vi "Acquire.vi"(8 "error in (no error)":errorcluster, 9 "Data Queue":refnum<queue>, 10 "Data Notifier":refnum<notifier>, 11 "Hardware Resources in":T1={"VISA resource name"="", "DAQ Type"=0, "Channel 1"={"Acquiring"=FALSE, "Enabled"=FALSE, "Terminal configuration"=32767, "Range"=0, "Coupling"=0}, "Channel 2"={"Acquiring"=FALSE, "Enabled"=FALSE, "Terminal configuration"=0, "Range"=0, "Coupling"=0}, "Timing"={"Sample Time [Time Units]"=0, "Actual Sample Time [s]"=0.0, "Samples per Iteration"=0, "Sample Clock Source"=0, "Time Units"=0, "t0"=timestamp(0 s since 1904-01-01)}, "PS Parameters"={"PS handle"=0, "PS Max_adc"=32767, "PS Enabled Array"=[], "PS Device Info"={"Driver Version"="", "USB Version"="", "Hardware"="", "Variant"="", "Batch and Serial"="", "Cal Date"="", "Kernel Version"="", "Digital HW Version"="", "Analogue HW Version"="", "Firmware 1"="", "Firmware 2"="", "MSO"=FALSE, "Number of Channels"=0}, "Channel 1 Buffer"=refnum, "Channel 2 Buffer"=refnum, "Resolution"=0, "USB Power"=FALSE}, "Trigger"={"Direction"=0, "Threshold [V]"=0.0, "Enabled"=FALSE, "Trigger Source"=0}, "Keithley Parameters"={"Previous End / Current Start"=0, "Quantity"=0}} {"Keithley Parameters"."Quantity" items=["Current", "Voltage"]; "Trigger"."Trigger Source" items=["Channel 1"=0, "Channel 2"=1, "Ext."=4]; "Trigger"."Direction" items=["Falling", "Rising"]; "PS Parameters"."Resolution" items=["8", "12", "14", "15", "16"]; "Timing"."Time Units" items=["Seconds"]; "Timing"."Sample Clock Source" items=["Internal", "External"]; "Channel 2"."Coupling" items=["AC", "DC"]; "Channel 2"."Range" items=["0.01", "0.02", "0.05", "0.1", "0.2", "0.5", "1", "2", "5", "10", "20", "50", "100", "1000"]; "Channel 2"."Terminal configuration" items=["Referenced Single Ended", "Differential"]; "Channel 1"."Coupling" items=["AC", "DC"]; "Channel 1"."Range" items=["0.01", "0.02", "0.05", "0.1", "0.2", "0.5", "1", "2", "5", "10", "20", "50", "100", "1000"]; "Channel 1"."Terminal configuration" items=["Referenced Single Ended", "Differential"]; "DAQ Type" items=["Simulated", "Tektronics DPO2k/3k/4k", "PicoScope 2000a Series", "Keithley DMM7510", "PicoScope 5000a Series"]}) -> (0 "error out":errorcluster, 3 "Hardware Resources out":T1={"VISA resource name"="", "DAQ Type"=0, "Channel 1"={"Acquiring"=FALSE, "Enabled"=FALSE, "Terminal configuration"=32767, "Range"=0, "Coupling"=0}, "Channel 2"={"Acquiring"=FALSE, "Enabled"=FALSE, "Terminal configuration"=0, "Range"=0, "Coupling"=0}, "Timing"={"Sample Time [Time Units]"=0, "Actual Sample Time [s]"=0.0, "Samples per Iteration"=0, "Sample Clock Source"=0, "Time Units"=0, "t0"=timestamp(0 s since 1904-01-01)}, "PS Parameters"={"PS handle"=0, "PS Max_adc"=32767, "PS Enabled Array"=[], "PS Device Info"={"Driver Version"="", "USB Version"="", "Hardware"="", "Variant"="", "Batch and Serial"="", "Cal Date"="", "Kernel Version"="", "Digital HW Version"="", "Analogue HW Version"="", "Firmware 1"="", "Firmware 2"="", "MSO"=FALSE, "Number of Channels"=0}, "Channel 1 Buffer"=refnum, "Channel 2 Buffer"=refnum, "Resolution"=0, "USB Power"=FALSE}, "Trigger"={"Direction"=0, "Threshold [V]"=0.0, "Enabled"=FALSE, "Trigger Source"=0}, "Keithley Parameters"={"Previous End / Current Start"=0, "Quantity"=0}} {"Keithley Parameters"."Quantity" items=["Current", "Voltage"]; "Trigger"."Trigger Source" items=["Channel 1"=0, "Channel 2"=1, "Ext."=4]; "Trigger"."Direction" items=["Falling", "Rising"]; "PS Parameters"."Resolution" items=["8", "12", "14", "15", "16"]; "Timing"."Time Units" items=["Seconds"]; "Timing"."Sample Clock Source" items=["Internal", "External"]; "Channel 2"."Coupling" items=["AC", "DC"]; "Channel 2"."Range" items=["0.01", "0.02", "0.05", "0.1", "0.2", "0.5", "1", "2", "5", "10", "20", "50", "100", "1000"]; "Channel 2"."Terminal configuration" items=["Referenced Single Ended", "Differential"]; "Channel 1"."Coupling" items=["AC", "DC"]; "Channel 1"."Range" items=["0.01", "0.02", "0.05", "0.1", "0.2", "0.5", "1", "2", "5", "10", "20", "50", "100", "1000"]; "Channel 1"."Terminal configuration" items=["Referenced Single Ended", "Differential"]; "DAQ Type" items=["Simulated", "Tektronics DPO2k/3k/4k", "PicoScope 2000a Series", "Keithley DMM7510", "PicoScope 5000a Series"]})   [LabVIEW 2016, in "Acquisition.lvlib"]
doc: "Perform the acquisition. Replace the contents of this diagram with calls to acquisition hardware."
uses:
  Acquisition.lvlib
  Hardware Configuration.ctl
  Signal Type.ctl
  Settings/Terminal Configuration.ctl
  Settings/Range.ctl
  Settings/Coupling.ctl
  Settings/Sampling Clock Source.ctl
  Settings/Time Units.ctl
  Settings/Resolution.ctl
  Settings/Trigger Direction.ctl
  Settings/Trigger Source.ctl
  Settings/Quantity.ctl
  support/Active channels.vi
  Settings/Settings.lvlib
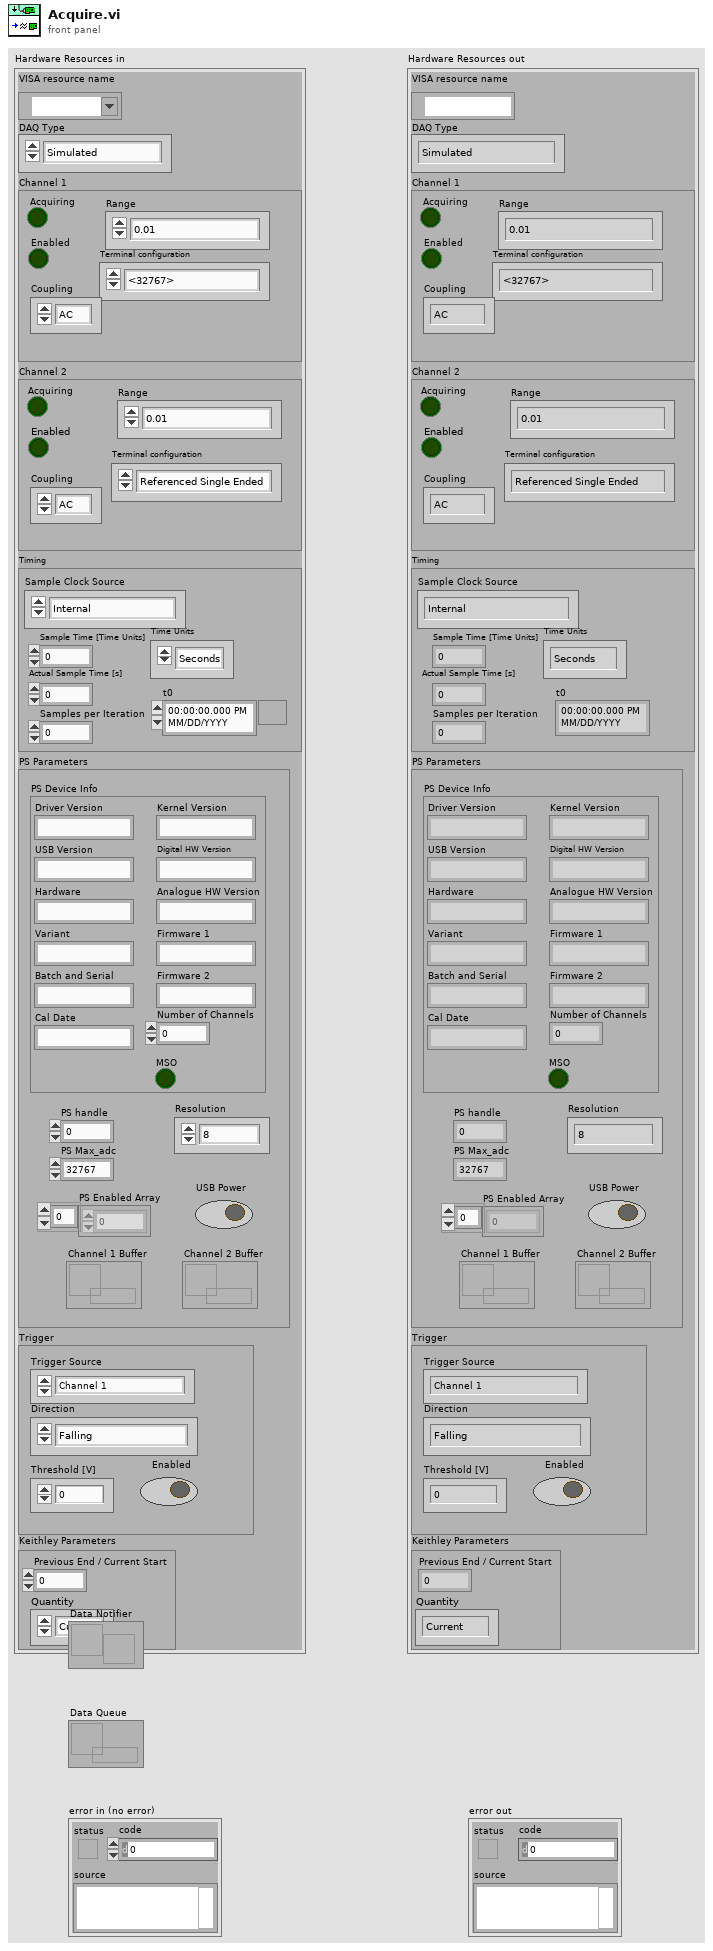
[diagram p1: front panel]
types:
  T1 = typedef "Acquisition.lvlib/Hardware Configuration.ctl" = cluster{"VISA resource name":refnum<visa-resource-name>, "DAQ Type":T2, "Channel 1":cluster{"Acquiring":bool, "Enabled":bool, "Terminal configuration":T3, "Range":T4, "Coupling":T5}, "Channel 2":cluster{"Acquiring":bool, "Enabled":bool, "Terminal configuration":T3, "Range":T4, "Coupling":T5}, "Timing":cluster{"Sample Time [Time Units]":u32, "Actual Sample Time [s]":dbl, "Samples per Iteration":u32, "Sample Clock Source":T6, "Time Units":T7, "t0":timestamp}, "PS Parameters":cluster{"PS handle":i16, "PS Max_adc":i16, "PS Enabled Array":i16[], "PS Device Info":cluster{"Driver Version":string, "USB Version":string, "Hardware":string, "Variant":string, "Batch and Serial":string, "Cal Date":string, "Kernel Version":string, "Digital HW Version":string, "Analogue HW Version":string, "Firmware 1":string, "Firmware 2":string, "MSO":bool, "Number of Channels":i16}, "Channel 1 Buffer":refnum<data-value>, "Channel 2 Buffer":refnum<data-value>, "Resolution":T8, "USB Power":bool}, "Trigger":cluster{"Direction":T9, "Threshold [V]":dbl, "Enabled":bool, "Trigger Source":T10}, "Keithley Parameters":cluster{"Previous End / Current Start":i32, "Quantity":T11}}
  T2 = typedef "Acquisition.lvlib/Signal Type.ctl" = u16
  T3 = typedef "Settings.lvlib/Terminal Configuration.ctl" = u16
  T4 = typedef "Settings.lvlib/Range.ctl" = u16
  T5 = typedef "Settings.lvlib/Coupling.ctl" = i16
  T6 = typedef "Settings.lvlib/Sampling Clock Source.ctl" = u16
  T7 = typedef "Settings.lvlib/Time Units.ctl" = u32
  T8 = typedef "Settings.lvlib/Resolution.ctl" = i32
  T9 = typedef "Settings.lvlib/Trigger Direction.ctl" = u16
  T10 = typedef "Settings.lvlib/Trigger Source.ctl" = u16
  T11 = typedef "Settings.lvlib/Quantity.ctl" = u16
  T12 = cluster{"PS handle":i16, "PS Max_adc":i16, "PS Enabled Array":i16[], "PS Device Info":cluster{"Driver Version":string, "USB Version":string, "Hardware":string, "Variant":string, "Batch and Serial":string, "Cal Date":string, "Kernel Version":string, "Digital HW Version":string, "Analogue HW Version":string, "Firmware 1":string, "Firmware 2":string, "MSO":bool, "Number of Channels":i16}, "Channel 1 Buffer":refnum<data-value>, "Channel 2 Buffer":refnum<data-value>, "Resolution":T8, "USB Power":bool}
  T13 = cluster{"Previous End / Current Start":i32, "Quantity":T11}
  T14 = cluster{"Acquiring":bool, "Enabled":bool, "Terminal configuration":T3, "Range":T4, "Coupling":T5}
  T15 = cluster{"Sample Time [Time Units]":u32, "Actual Sample Time [s]":dbl, "Samples per Iteration":u32, "Sample Clock Source":T6, "Time Units":T7, "t0":timestamp}
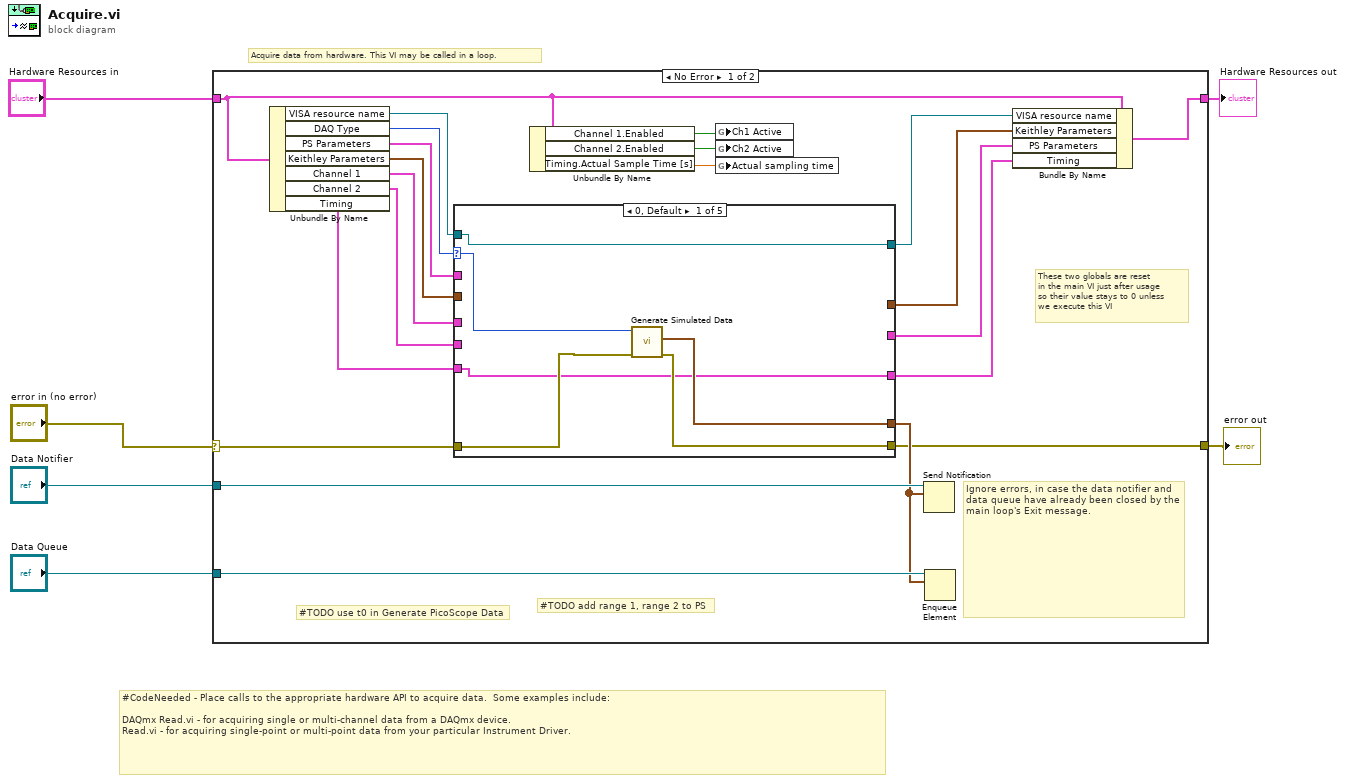
[diagram p0: block diagram]
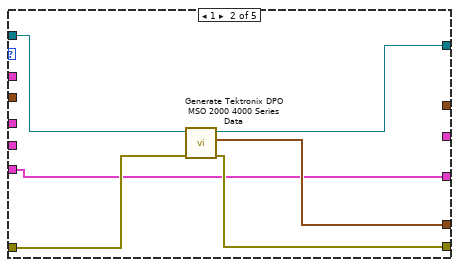
[diagram p2: hidden frame]
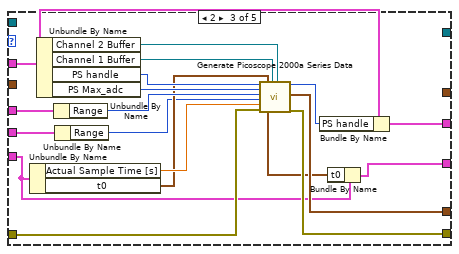
[diagram p3: hidden frame]
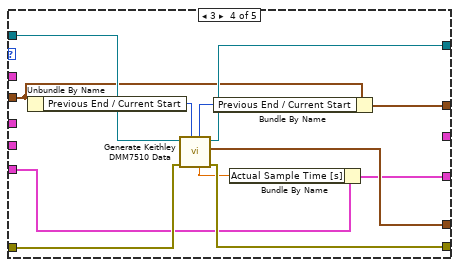
[diagram p4: hidden frame]
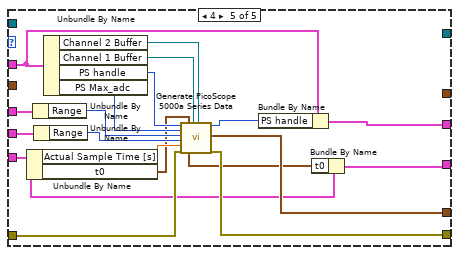
[diagram p5: hidden frame]
diagram:
  # "Acquire data from hardware. This VI may be called in a loop."
  # "#CodeNeeded - Place calls to the appropriate hardware API to acquire data.  Some examples include:\n\nDAQmx Read.vi - for acquiring single or multi-channel data from a DAQmx device.\nRead.vi - for acquiring single-point or multi-point data from your particular Instrument Driver."
  n1 = case shown="No Error" "error in (no error)" {
    selector: "error in (no error)" -> [w26 w90]
    tunnel: [w22 w90] -> w5
    tunnel: "Hardware Resources in" -> [w10 w91]
    tunnel: [w27 w91] -> w3
    tunnel: "Data Notifier" -> [w25 _]
    tunnel: "Data Queue" -> [w24 _]
    frame No Error {
      # "#TODO add range 1, range 2 to PS"
      # "These two globals are reset\nin the main VI just after usage\nso their value stays to 0 unless\nwe execute this VI"
      # "#TODO use t0 in Generate PicoScope Data"
      # "Ignore errors, in case the data notifier and data queue have already been closed by the main loop's Exit message."
      n2 = Unbundle By Name(w10) -> ("VISA resource name"=w20:refnum<visa-resource-name>, "DAQ Type"=w21:T2, "PS Parameters"=w15:T12, "Keithley Parameters"=w18:T13, "Channel 1"=w14:T14, "Channel 2"=w13:T14, "Timing"=w12:T15)
      n3 = case shown="0, Default" w21 {
        selector: w21 -> [w29 _ _ _ _]
        tunnel: w26 -> [w32 w39 w57 w69 w89]
        tunnel: [w30 w36 w53 w66 w87] -> w23
        tunnel: [w31 w38 w56 w67 w88] -> w22
        tunnel: w20 -> [w33 w37 _ w70 _]
        tunnel: [w33 w35 _ w68 _] -> w19
        tunnel: w18 -> [_ _ _ w64 _]
        tunnel: w15 -> [_ _ w55 _ w85]
        tunnel: w12 -> [w28 w34 w43 w61 w74]
        tunnel: [_ _ w58 _ w83] -> w17
        tunnel: [_ _ _ w62 _] -> w16
        tunnel: w14 -> [_ _ w48 _ w78]
        tunnel: w13 -> [_ _ w47 _ w76]
        tunnel: [w28 w34 w41 w59 w73] -> w11
        frame 0, Default {
          n4 = call "Generate Simulated Data.vi"("error in (no error)"=w32, "Signal Type"=w29) -> ("error out"=w31:errorcluster, "Graph Data"=w30:waveform(dbl)[])  [unwired: 8 in]
        }
        frame 1 {
          n5 = call "Generate Tektronix DPO MSO 2000 4000 Series Data.vi"("error in (no error)"=w39, "VISA resource name"=w37) -> ("error out"=w38:errorcluster, "Graph Data"=w36:waveform(dbl)[], "VISA resource name 2"=w35:refnum<visa-resource-name>)  [unwired: 7 in]
        }
        frame 2 {
          n6 = Unbundle By Name(w43) -> ("Actual Sample Time [s]"=w45:dbl, "t0"=w44:timestamp)
          n7 = Unbundle By Name(w55) -> ("Channel 2 Buffer"=w52:refnum<data-value>, "Channel 1 Buffer"=w51:refnum<data-value>, "PS handle"=w50:i16, "PS Max_adc"=w49:i16)
          n8 = Unbundle By Name(w48) -> ("Range"=w46:T4)
          n9 = Unbundle By Name(w47) -> ("Range"=w40:T4)
          n10 = call "Generate Picoscope 2000a Series Data.vi"("handle in"=w50, "Max ADC"=w49, "Ch1 Range Index"=w46, "Ch2 Range Index"=w40, "Actual Sample Interval"=w45, "error in (no error)"=w57, "t0"=w44, "Channel 1 Buff In"=w51, "Channel 2 Buff In"=w52) -> ("next t0"=w42:timestamp, "handle out"=w54:i16, "Graph Data"=w53:waveform(dbl)[], "error out"=w56:errorcluster)  [unwired: 5 in, 2 out]
          n11 = Bundle By Name(cluster=w55, "PS handle"=w54) -> (w58:T12)
          n12 = Bundle By Name(cluster=w43, "t0"=w42) -> (w41:T15)
        }
        frame 3 {
          n13 = Unbundle By Name(w64) -> ("Previous End / Current Start"=w65:i32)
          n14 = call "Generate Keithley DMM7510 Data.vi"("Previous End"=w65, "error in (no error)"=w69, "VISA resource name in"=w70) -> ("error out"=w67:errorcluster, "Graph Data"=w66:waveform(dbl)[], "VISA resource name out"=w68:refnum<visa-resource-name>, "Actual sampling time (mean)"=w60:dbl, "Current End"=w63:i32)  [unwired: 4 in]
          n15 = Bundle By Name(cluster=w64, "Previous End / Current Start"=w63) -> (w62:T13)
          n16 = Bundle By Name(cluster=w61, "Actual Sample Time [s]"=w60) -> (w59:T15)
        }
        frame 4 {
          n17 = Unbundle By Name(w74) -> ("Actual Sample Time [s]"=w86:dbl, "t0"=w72:timestamp)
          n18 = Unbundle By Name(w78) -> ("Range"=w77:T4)
          n19 = Unbundle By Name(w76) -> ("Range"=w75:T4)
          n20 = Unbundle By Name(w85) -> ("Channel 2 Buffer"=w81:refnum<data-value>, "Channel 1 Buffer"=w82:refnum<data-value>, "PS handle"=w80:i16, "PS Max_adc"=w79:i16)
          n21 = call "Generate PicoScope 5000a Series Data.vi"("handle in"=w80, "Max ADC"=w79, "Ch1 Range Index"=w77, "Ch2 Range Index"=w75, "Actual Sample Interval"=w86, "error in (no error)"=w89, "t0"=w72, "Channel 1 Buff In"=w82, "Channel 2 Buff In"=w81) -> ("next t0"=w71:timestamp, "handle out"=w84:i16, "Graph Data"=w87:waveform(dbl)[], "error out"=w88:errorcluster)  [unwired: 5 in, 2 out]
          n22 = Bundle By Name(cluster=w85, "PS handle"=w84) -> (w83:T12)
          n23 = Bundle By Name(cluster=w74, "t0"=w71) -> (w73:T15)
        }
      }
      n24 = Unbundle By Name(w10) -> ("Channel 1.Enabled"=w9:bool, "Channel 2.Enabled"=w7:bool, "Timing.Actual Sample Time [s]"=w8:dbl)
      n25 = global write "Active channels.vi" "Ch1 Active"(w9) -> ()
      n26 = global write "Active channels.vi" "Ch2 Active"(w7) -> ()
      n27 = global write "Active channels.vi" "Actual sampling time"(w8) -> ()
      n28 = Send Notification(notification=w23, notifier=w25) -> ()  [unwired: 1 in, 2 out]
      n29 = Enqueue Element(queue=w24, element=w23) -> ()  [unwired: 2 in, 3 out]
      n30 = Bundle By Name(cluster=w10, "VISA resource name"=w19, "Keithley Parameters"=w16, "PS Parameters"=w17, "Timing"=w11) -> (w27:T1)
    }
    frame Error {
    }
  }
  "Hardware Resources out" <- w3
  "error out" <- w5
